vi "FK.vi"(8 "error in (no error)":errorcluster, 10 "joints":dbl[](array[numeric]), 11 "Delta Robot Kinematics in":refnum<class "Delta Robot Kinematics.lvclass">) -> (0 "error out":errorcluster, 1 "exist":bool, 2 "p":dbl[](array[numeric]), 3 "Delta Robot Kinematics out":refnum<class "Delta Robot Kinematics.lvclass">)   [LabVIEW 2013, in "Delta Robot Kinematics.lvclass"]
uses:
  Delta Robot Kinematics.lvclass
  Delta Robot Kinematics.lvclass/Delta Robot Kinematics.ctl
  <vilib>/Analysis/baseanly.llb/A x Vector.vi
  <vilib>/Analysis/_algsub.llb/Real Vector Norm.vi
  <vilib>/Analysis/baseanly.llb/Outer Product.vi
  <vilib>/Analysis/baseanly.llb/Real Outer Product.vi
  <vilib>/robotics/Kinematics/Create Lie Group Matrix.vi
  <vilib>/Analysis/7linalg.llb/Create Special Matrix.vi
  <vilib>/Analysis/7linalg.llb/Create Special Real Matrix.vi
  <vilib>/Analysis/Matrix/Numeric/Multiply/Multiply.vi
  <vilib>/Analysis/Matrix/Numeric/Multiply/Multiply - RM,R.vi
  <vilib>/Analysis/Matrix/Numeric/Multiply/Multiply - R,RM.vi
  <vilib>/Analysis/Matrix/Numeric/Add/Add.vi
  <vilib>/Analysis/Matrix/Numeric/Add/Add - RM,RM.vi
  <vilib>/robotics/Kinematics/NI_Kinematics.lvlib
  <vilib>/Analysis/NI_AALBase.lvlib
  <vilib>/Analysis/NI_AALPro.lvlib
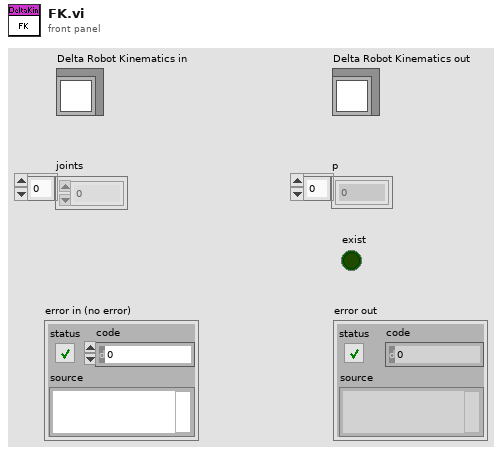
[diagram p1: front panel]
types:
  T1 = typedef "NI_Matrix.lvlib/RealMatrix.ctl" = dbl[][]
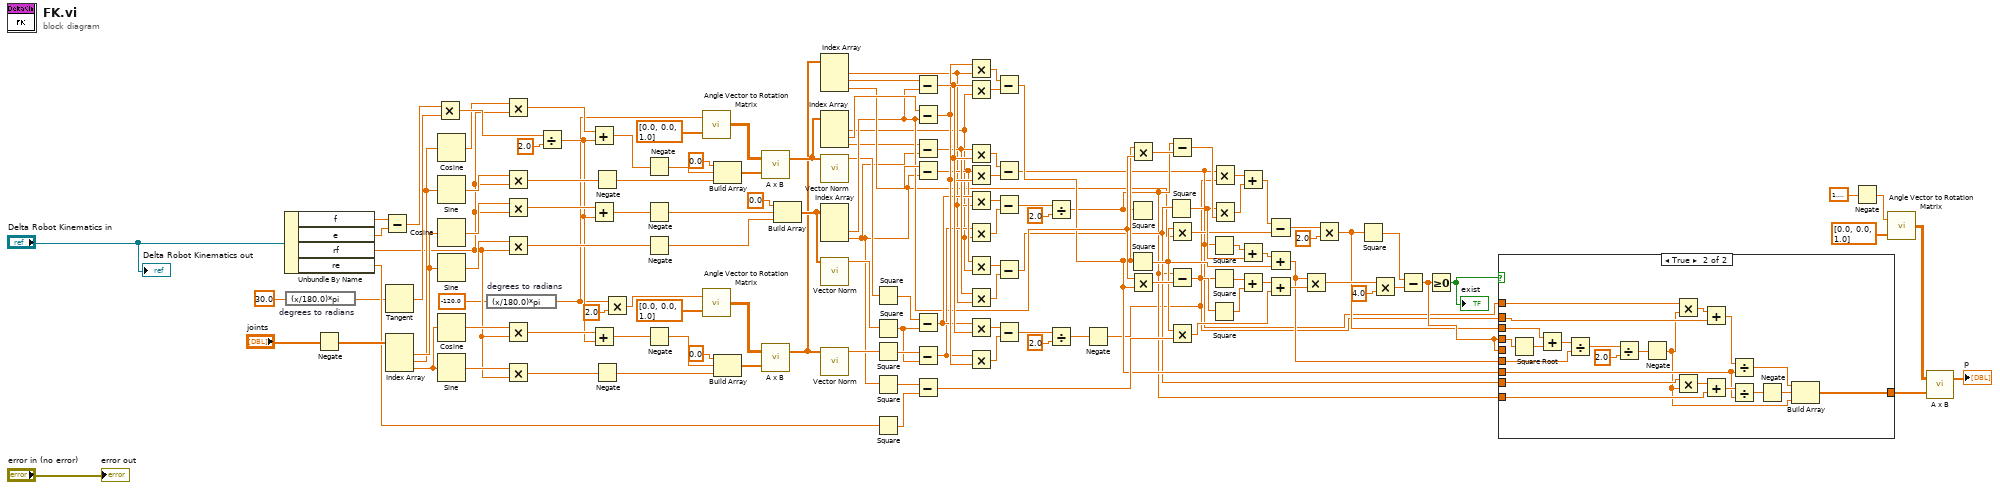
[diagram p0: block diagram]
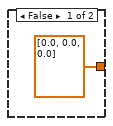
[diagram p2: hidden frame]
diagram:
  n1 = Unbundle By Name("Delta Robot Kinematics in") -> ("f"=w9:dbl, "e"=w8:dbl, "rf"=w7:dbl, "re"=w6:dbl)
  n2 = expression code="(x/180.0)*pi" "degrees to radians"(30.0) -> (w4:dbl)
  n3 = Negate(x="joints") -> (-x=w31:dbl[])
  n4 = Subtract(x=w9, y=w8) -> (x-y=w130:dbl)
  n5 = Tangent(1:w4) -> (0:w129:dbl)
  n6 = Index Array(array=w31) -> (element #1=w123:dbl, element #2=w52:dbl, element #3=w51:dbl)  [unwired: 3 in]
  n7 = Multiply(x=w130, y=w129) -> (x*y=w128:dbl)
  n8 = Cosine(x=w52) -> (cos(x)=w38:dbl)
  n9 = Sine(x=w52) -> (sin(x)=w36:dbl)
  n10 = Cosine(x=w123) -> (cos(x)=w126:dbl)
  n11 = Sine(x=w123) -> (sin(x)=w122:dbl)
  n12 = Cosine(x=w51) -> (cos(x)=w37:dbl)
  n13 = Sine(x=w51) -> (sin(x)=w34:dbl)
  n14 = expression code="(x/180.0)*pi" "degrees to radians"(-120.0) -> (w2:dbl)
  n15 = Multiply(x=w38, y=w7) -> (x*y=w50:dbl)
  n16 = Multiply(x=w36, y=w7) -> (x*y=w48:dbl)
  n17 = Multiply(x=w126, y=w7) -> (x*y=w125:dbl)
  n18 = Multiply(x=w122, y=w7) -> (x*y=w121:dbl)
  n19 = Multiply(x=w37, y=w7) -> (x*y=w39:dbl)
  n20 = Multiply(x=w34, y=w7) -> (x*y=w41:dbl)
  n21 = Divide(x=w128, y=2.0) -> (x/y=w35:dbl)
  n22 = Add(x=w50, y=w35) -> (x+y=w49:dbl)
  n23 = Add(x=w125, y=w35) -> (x+y=w124:dbl)
  n24 = Add(x=w39, y=w35) -> (x+y=w40:dbl)
  n25 = Negate(x=w48) -> (-x=w46:dbl)
  n26 = Negate(x=w41) -> (-x=w43:dbl)
  n27 = Multiply(x=w2, y=2.0) -> (x*y=w27:dbl)
  n28 = Negate(x=w49) -> (-x=w47:dbl)
  n29 = Negate(x=w124) -> (-x=w120:dbl)
  n30 = Negate(x=w121) -> (-x=w119:dbl)
  n31 = Negate(x=w40) -> (-x=w42:dbl)
  n32 = call <vilib>:"Angle Vector to Rotation Matrix.vi"("vector"=dbl[] [0.0, 0.0, 1.0], "angle"=w2) -> ("rotation matrix"=w116:T1)
  n33 = call <vilib>:"Angle Vector to Rotation Matrix.vi"("vector"=dbl[] [0.0, 0.0, 1.0], "angle"=w27) -> ("rotation matrix"=w29:T1)
  n34 = Build Array(0.0 ("element"), w47, w46) -> (w33:dbl[])
  n35 = Build Array(0.0 ("element"), w42, w43) -> (w32:dbl[])
  n36 = call-poly <vilib>:"A x B.vi"("Vector"=w33, "A"=w116) -> ("A x Vector"=w110:dbl[])  [unwired: 1 out]
  n37 = call-poly <vilib>:"A x B.vi"("Vector"=w32, "A"=w29) -> ("A x Vector"=w109:dbl[])  [unwired: 1 out]
  n38 = Build Array(0.0 ("element"), w120, w119) -> (w111:dbl[])
  n39 = Index Array(array=w109) -> (element #1=w92:dbl, element #2=w113:dbl, element #3=w107:dbl)  [unwired: 3 in]
  n40 = Index Array(array=w110) -> (element #1=w19:dbl, element #2=w115:dbl, element #3=w20:dbl)  [unwired: 3 in]
  n41 = call-poly <vilib>:"Vector Norm.vi"("Input Vector"=w110) -> ("norm"=w24:dbl)  [unwired: 9 in, 1 out]
  n42 = Index Array(array=w111) -> (element #2=w77:dbl, element #3=w18:dbl)  [unwired: 3 in, 1 out]
  n43 = call-poly <vilib>:"Vector Norm.vi"("Input Vector"=w111) -> ("norm"=w22:dbl)  [unwired: 9 in, 1 out]
  n44 = call-poly <vilib>:"Vector Norm.vi"("Input Vector"=w109) -> ("norm"=w26:dbl)  [unwired: 9 in, 1 out]
  n45 = Square(x=w24) -> (x^2=w23:dbl)
  n46 = Square(x=w22) -> (x^2=w21:dbl)
  n47 = Square(x=w26) -> (x^2=w25:dbl)
  n48 = Square(x=w18) -> (x^2=w72:dbl)
  n49 = Square(x=w6) -> (x^2=w71:dbl)
  n50 = Subtract(x=w113, y=w77) -> (x-y=w105:dbl)
  n51 = Subtract(x=w115, y=w77) -> (x-y=w104:dbl)
  n52 = Subtract(x=w20, y=w18) -> (x-y=w98:dbl)
  n53 = Subtract(x=w107, y=w18) -> (x-y=w94:dbl)
  n54 = Subtract(x=w23, y=w21) -> (x-y=w95:dbl)
  n55 = Subtract(x=w25, y=w21) -> (x-y=w93:dbl)
  n56 = Subtract(x=w72, y=w71) -> (x-y=w70:dbl)
  n57 = Multiply(x=w104, y=w92) -> (x*y=w114:dbl)
  n58 = Multiply(x=w105, y=w19) -> (x*y=w112:dbl)
  n59 = Multiply(x=w98, y=w105) -> (x*y=w108:dbl)
  n60 = Multiply(x=w94, y=w104) -> (x*y=w106:dbl)
  n61 = Multiply(x=w95, y=w92) -> (x*y=w91:dbl)
  n62 = Multiply(x=w93, y=w19) -> (x*y=w90:dbl)
  n63 = Multiply(x=w94, y=w19) -> (x*y=w97:dbl)
  n64 = Multiply(x=w98, y=w92) -> (x*y=w96:dbl)
  n65 = Multiply(x=w95, y=w105) -> (x*y=w103:dbl)
  n66 = Multiply(x=w93, y=w104) -> (x*y=w102:dbl)
  n67 = Subtract(x=w114, y=w112) -> (x-y=w61:dbl)
  n68 = Subtract(x=w108, y=w106) -> (x-y=w17:dbl)
  n69 = Subtract(x=w91, y=w90) -> (x-y=w89:dbl)
  n70 = Subtract(x=w97, y=w96) -> (x-y=w60:dbl)
  n71 = Subtract(x=w103, y=w102) -> (x-y=w101:dbl)
  n72 = Divide(x=w89, y=2.0) -> (x/y=w59:dbl)
  n73 = Divide(x=w101, y=2.0) -> (x/y=w99:dbl)
  n74 = Negate(x=w99) -> (-x=w16:dbl)
  n75 = Square(x=w59) -> ()  [unwired: 1 out]
  n76 = Square(x=w61) -> (x^2=w69:dbl)
  n77 = Multiply(x=w61, y=w77) -> (x*y=w85:dbl)
  n78 = Multiply(x=w77, y=w61) -> (x*y=w76:dbl)
  n79 = Square(x=w60) -> (x^2=w83:dbl)
  n80 = Subtract(x=w59, y=w85) -> (x-y=w84:dbl)
  n81 = Multiply(x=w69, y=w18) -> (x*y=w80:dbl)
  n82 = Subtract(x=w59, y=w76) -> (x-y=w75:dbl)
  n83 = Multiply(x=w69, y=w70) -> (x*y=w67:dbl)
  n84 = Square(x=w17) -> (x^2=w87:dbl)
  n85 = Square(x=w16) -> (x^2=w74:dbl)
  n86 = Square(x=w75) -> (x^2=w73:dbl)
  n87 = Multiply(x=w17, y=w16) -> (x*y=w15:dbl)
  n88 = Multiply(x=w83, y=w84) -> (x*y=w82:dbl)
  n89 = Add(x=w15, y=w82) -> (x+y=w81:dbl)
  n90 = Add(x=w87, y=w83) -> (x+y=w86:dbl)
  n91 = Add(x=w74, y=w73) -> (x+y=w68:dbl)
  n92 = Subtract(x=w81, y=w80) -> (x-y=w79:dbl)
  n93 = Add(x=w86, y=w69) -> (x+y=w56:dbl)
  n94 = Add(x=w68, y=w67) -> (x+y=w66:dbl)
  n95 = Multiply(x=w56, y=w66) -> (x*y=w65:dbl)
  n96 = Multiply(x=w79, y=2.0) -> (x*y=w57:dbl)
  n97 = Square(x=w57) -> (x^2=w63:dbl)
  n98 = Multiply(x=w65, y=4.0) -> (x*y=w62:dbl)
  n99 = Subtract(x=w63, y=w62) -> (x-y=w58:dbl)
  n100 = Greater Or Equal To 0?(x=w58) -> (x >= 0?=w11:bool)
  "exist" <- w11
  n101 = case shown="True" w11 {
    tunnel: w58 -> [_ _]
    tunnel: w17 -> [_ w154]
    tunnel: w16 -> [_ w152]
    tunnel: w61 -> [_ w146]
    tunnel: w60 -> [_ w150]
    tunnel: w59 -> [_ w148]
    tunnel: w58 -> [_ w145]
    tunnel: w57 -> [_ w143]
    tunnel: w56 -> [_ w141]
    tunnel: [dbl[] [0.0, 0.0, 0.0] w138] -> w53
    frame False {
    }
    frame True {
      n102 = Square Root(x=w145) -> (sqrt(x)=w144:dbl)
      n103 = Add(x=w143, y=w144) -> (x+y=w142:dbl)
      n104 = Divide(x=w142, y=w141) -> (x/y=w140:dbl)
      n105 = Divide(x=w140, y=2.0) -> (x/y=w137:dbl)
      n106 = Negate(x=w137) -> (-x=w136:dbl)
      n107 = Multiply(x=w154, y=w136) -> (x*y=w153:dbl)
      n108 = Multiply(x=w150, y=w136) -> (x*y=w149:dbl)
      n109 = Add(x=w153, y=w152) -> (x+y=w151:dbl)
      n110 = Add(x=w149, y=w148) -> (x+y=w147:dbl)
      n111 = Divide(x=w151, y=w146) -> (x/y=w135:dbl)
      n112 = Divide(x=w147, y=w146) -> (x/y=w134:dbl)
      n113 = Negate(x=w134) -> (-x=w133:dbl)
      n114 = Build Array(w135, w133, w136) -> (w138:dbl[])
    }
  }
  n115 = Negate(x=1.5707963267948966) -> (-x=w13:dbl)
  n116 = call <vilib>:"Angle Vector to Rotation Matrix.vi"("vector"=dbl[] [0.0, 0.0, 1.0], "angle"=w13) -> ("rotation matrix"=w54:T1)
  n117 = call-poly <vilib>:"A x B.vi"("Vector"=w53, "A"=w54) -> ("A x Vector"=→"p":dbl[])  [unwired: 1 out]
  "Delta Robot Kinematics out" <- "Delta Robot Kinematics in"
  "error out" <- "error in (no error)"
